vi "Trigger Update Dynamic.vi"(1 "Trigger":bool) -> (0 "Update":bool)   [LabVIEW 2018]
uses:
  <vilib>/Rock Robotics/WPI/DriverStation/WPI_DriverStationRobotMode2.ctl
  Robot Global Data.vi
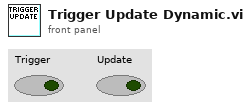
[diagram p1: front panel]
types:
  T1 = typedef "WPI_DriverStationRobotMode2.ctl" = enum16{"Autonomous Disabled", "Autonomous Enabled", "Teleop Disabled", "Teleop Enabled", "Disconnected", "Finish", "Test Disabled", "Test Enabled", "Emergency Stopped"}
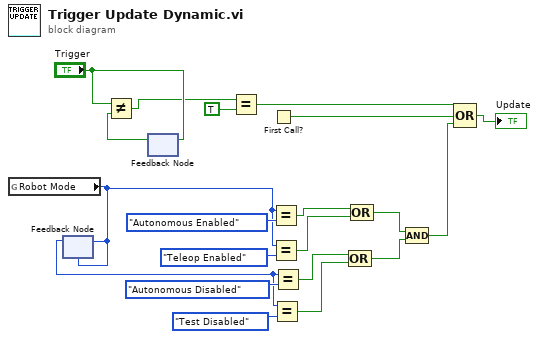
[diagram p0: block diagram]
diagram:
  n1 = global read "Robot Global Data.vi" "Robot Mode"() -> (w9:T1)
  n2 = feedback #1(w9) -> (w8:T1)
  n3 = feedback-in #1(w9) -> ()
  n4 = feedback-in #2("Trigger") -> ()
  n5 = feedback #2() -> (w20:bool)  [unwired: 1 in]
  n6 = Not Equal?(x="Trigger", y=w20) -> (x != y?=w18:bool)
  n7 = Equal?(x=w18, y=TRUE) -> (x = y?=w15:bool)
  n8 = First Call?() -> (First Call?: T/F=w14:bool)
  n9 = Equal?(x=w9, y=WPI_DriverStationRobotMode2."Autonomous Enabled") -> (x = y?=w7:bool)
  n10 = Equal?(x=w9, y=WPI_DriverStationRobotMode2."Teleop Enabled") -> (x = y?=w6:bool)
  n11 = Equal?(x=w8, y=WPI_DriverStationRobotMode2."Test Disabled") -> (x = y?=w4:bool)
  n12 = Equal?(x=w8, y=WPI_DriverStationRobotMode2."Autonomous Disabled") -> (x = y?=w5:bool)
  n13 = Compound Arithmetic op=OR(w5, w4) -> (w2:bool)
  n14 = Compound Arithmetic op=OR(w7, w6) -> (w3:bool)
  n15 = Compound Arithmetic op=AND(w3, w2) -> (w1:bool)
  n16 = Compound Arithmetic op=OR(w15, w14, w1) -> (→"Update":bool)
